vi "PRL STR Get Selected Indices.vi"(10 "Selected":string[](array[string]), 11 "All":string[](array[string])) -> (3 "Indices":i32[](array[numeric]))   [LabVIEW 2013, in "PMU Recorder Light.lvlib"]
uses:
  PMU Recorder Light.lvlib
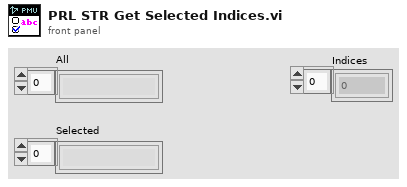
[diagram p1: front panel]
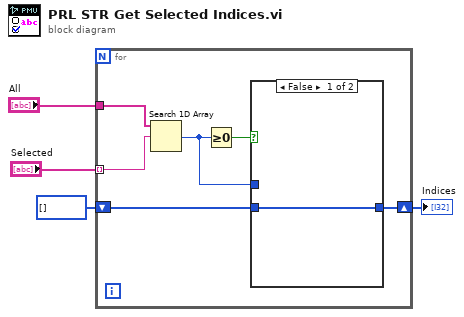
[diagram p0: block diagram]
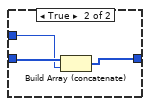
[diagram p2: hidden frame]
diagram:
  n1 = for {
    tunnel: "All" -> [w10]
    tunnel: "Selected" -> [w9] mode=indexing
    shift-right: [w5] -> w1
    shift-left: i32[] [] -> [w6]
    n2 = Search 1D Array(1D array=w10, element=w9) -> (index of element=w7:i32)  [unwired: 1 in]
    n3 = Greater Or Equal To 0?(x=w7) -> (x >= 0?=w8:bool)
    n4 = case shown="False" w8 {
      tunnel: w7 -> [_ w13]
      tunnel: w6 -> [w11 w14]
      tunnel: [w11 w12] -> w5
      frame False {
      }
      frame True {
        n5 = Build Array (concatenate)(w14, w13) -> (w12:i32[])
      }
    }
  }
  "Indices" <- w1
